vi "IntegraMeter_Initialize.vi"(8 "error in":errorcluster, 11 "VISA resource name":refnum<visa-resource-name>) -> (0 "error out":errorcluster, 3 "VISA resource name out":refnum<visa-resource-name>)   [LabVIEW 2024]
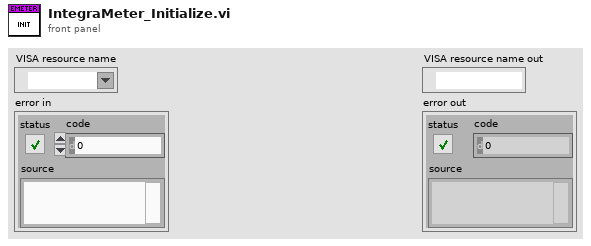
[diagram p1: front panel]
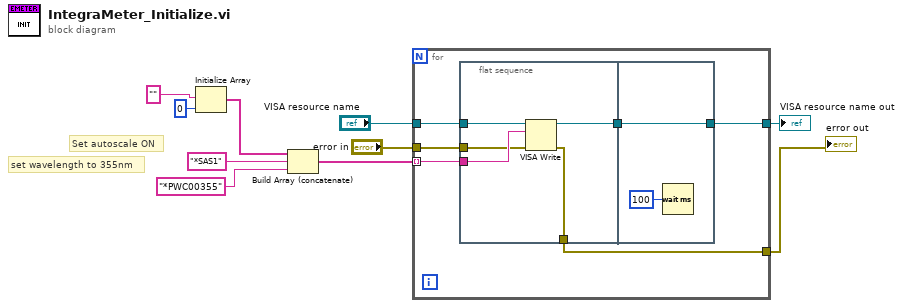
[diagram p0: block diagram]
diagram:
  # "set wavelength to 355nm"
  # "Set autoscale ON"
  n1 = Initialize Array("", 0 ("dimension size")) -> (w6:string[])
  n2 = Build Array (concatenate)(w6, "*SAS1", "*PWC00355") -> (w3:string[])
  n3 = for {
    tunnel: "VISA resource name" -> [w16]
    tunnel: [w15] -> w9
    tunnel: w3 -> [w13] mode=indexing
    tunnel: "error in" -> [w12]
    tunnel: [w11] -> w1
    n4 = flat-sequence {
      tunnel: w16 -> [w21]
      tunnel: [w20] -> w14
      tunnel: w13 -> [w19]
      tunnel: w12 -> [w18]
      tunnel: [w17] -> w11
      tunnel: [w22] -> w15
      tunnel: w14 -> [w22]
      frame #0 {
        n5 = VISA Write(VISA resource name=w21, write buffer=w19, error in (no error)=w18) -> (VISA resource name out=w20:refnum<visa-resource-name>, error out=w17:errorcluster)  [unwired: 1 out]
      }
      frame #1 {
        n6 = Wait (ms)(milliseconds to wait=u32 100) -> ()  [unwired: 1 out]
      }
    }
  }
  "VISA resource name out" <- w9
  "error out" <- w1
